vi "FlatToRichni_measurementlink_pinmap_v1_PinMap.vi"(5 "OutputClusterType":T1, 11 "InputCluster":T2) -> (3 "OutputCluster":T1)   [LabVIEW 2020, in "ni.measurementlink.pinmap.v1.lvlib"]
uses:
  ni.measurementlink.pinmap.v1.lvlib
  ni_measurementlink_pinmap_v1_PinMap.ctl
  ni_measurementlink_pinmap_v1_PinMap_Flat.ctl
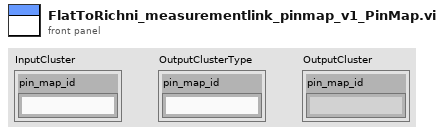
[diagram p1: front panel]
types:
  T1 = typedef "ni.measurementlink.pinmap.v1.lvlib/ni_measurementlink_pinmap_v1_PinMap.ctl" = cluster{"pin_map_id":string}
  T2 = typedef "ni.measurementlink.pinmap.v1.lvlib/ni_measurementlink_pinmap_v1_PinMap_Flat.ctl" = cluster{"pin_map_id":string}
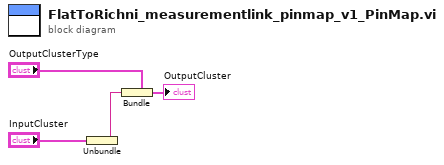
[diagram p0: block diagram]
diagram:
  n1 = Unbundle "Unbundle"("InputCluster") -> ("pin_map_id"=w1:string)
  n2 = Bundle "Bundle"(cluster="OutputClusterType", "pin_map_id"=w1) -> (→"OutputCluster":T1)
